vi "Device.GetPublicEventsRegistration.vi"(8 "error in (no error)":errorcluster, 11 "Device in":refnum<class "Device.lvclass">) -> (0 "error out":errorcluster, 2 "Device Public Events":refnum<event-registration>, 3 "Device out":refnum<class "Device.lvclass">)   [LabVIEW 2017, in "Device.lvclass"]
uses:
  Device.lvclass
  Typedefs/PublicEvents--Cluster.ctl
  Typedefs/PublicEvents--Device.Initialized.ctl
  Typedefs/PublicEvents--Device.Uninitialized.ctl
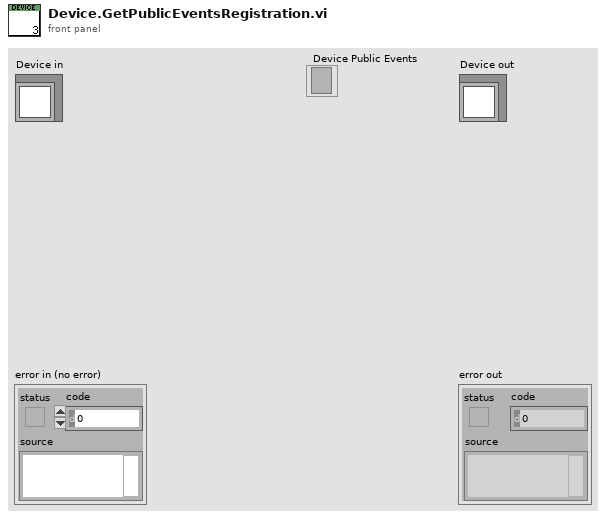
[diagram p1: front panel]
types:
  T1 = typedef "Device.lvclass/PublicEvents--Cluster.ctl" = cluster{"Initialized":refnum<user-event>, "Uninitialized":refnum<user-event>}
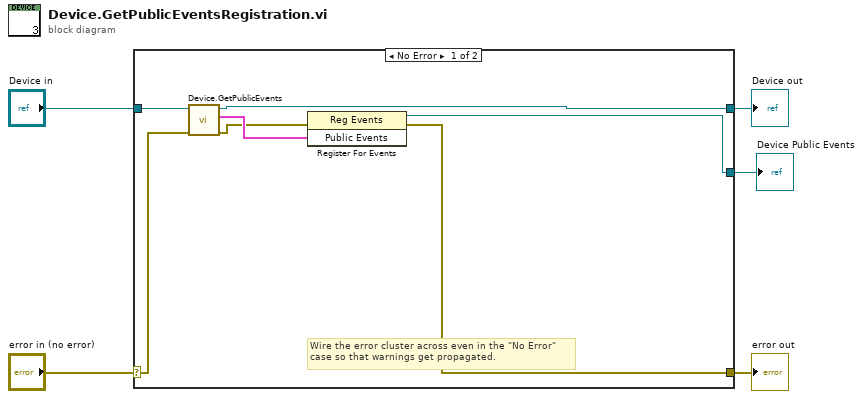
[diagram p0: block diagram]
diagram:
  n1 = case shown="No Error" "error in (no error)" {
    selector: "error in (no error)" -> [w11 w14]
    tunnel: [w7 w14] -> w4
    tunnel: [w8 w13] -> w2
    tunnel: "Device in" -> [w12 w13]
    tunnel: [w6 _] -> w1
    frame No Error {
      # "Wire the error cluster across even in the \"No Error\"\ncase so that warnings get propagated."
      n2 = call "Device.GetPublicEvents.vi"("error in (no error)"=w11, "Device in"=w12) -> ("error out"=w9:errorcluster, "Public Events"=w10:T1, "Device out"=w8:refnum<class "Device.lvclass">)  [unwired: 7 in]
      n3 = register-events(error in=w9, w10) -> (reference out=w6:refnum<event-registration>, error out=w7:errorcluster)  [unwired: 1 in]
    }
    frame Error {
    }
  }
  "error out" <- w4
  "Device out" <- w2
  "Device Public Events" <- w1
